vi "cw_4_4.vi"() -> ()   [LabVIEW 2022 SP3]
panel:
  out "reversed string":string
  in  "String":string
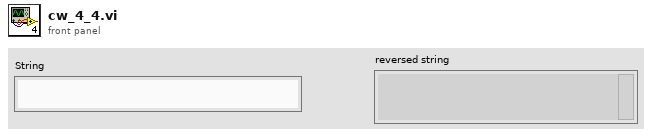
[diagram p1: front panel]
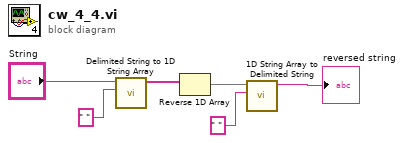
[diagram p0: block diagram]
diagram:
  n1 = call <vilib>:"Delimited String to 1D String Array.vi"("delimiter"=" ", "delimited string"="String") -> ("string array"=w4:string[])  [unwired: 9 in]
  n2 = Reverse 1D Array(array=w4) -> (reversed array=w3:string[])
  n3 = call <vilib>:"1D String Array to Delimited String.vi"("delimiter"=" ", "string array"=w3) -> ("delimited string"=→"reversed string":string)  [unwired: 9 in]
